vi "Init Msg Output.vi"() -> (3 "TEMPLATE Msg Output out":refnum<class "TEMPLATE Msg Output.lvclass">)   [LabVIEW 2025, in "_Template.lvlib" / "Templates.lvlib" / "TEMPLATE Msg.lvlib" / "TEMPLATE Msg Output.lvlib" / "TEMPLATE Msg Output.lvclass"]
uses:
  TEMPLATE Msg Output.lvclass
panel:
  # "This front panel should not be manipulated."
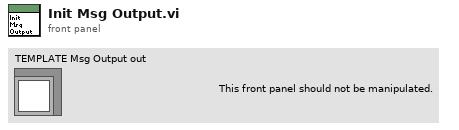
[diagram p1: front panel]
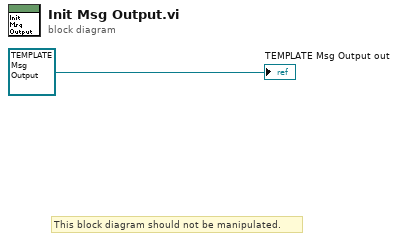
[diagram p0: block diagram]
diagram:
  # "This block diagram should not be manipulated."
  "TEMPLATE Msg Output out" <- refnum<class "TEMPLATE Msg Output.lvclass"> refnum ("Object")
